vi "Proba.vi"() -> ()   [LabVIEW 2013]
panel:
  out "ora":dbl
  in  "tsim [nap]":i32=7
  in  "h [s]":i32=60
  in  "rhoPCM":dbl=1100.0
  in  "Tbelsolevego_0":dbl=22.0
  in  "c_lev":dbl=1.0
  in  "rholevego":dbl=1.3
  in  "Vlevego":dbl=0.446
  in  "Top_felso":dbl=28.0
  in  "Top_also":dbl=24.0
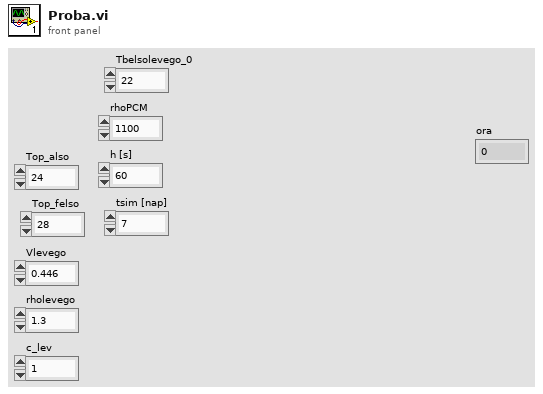
[diagram p1: front panel]
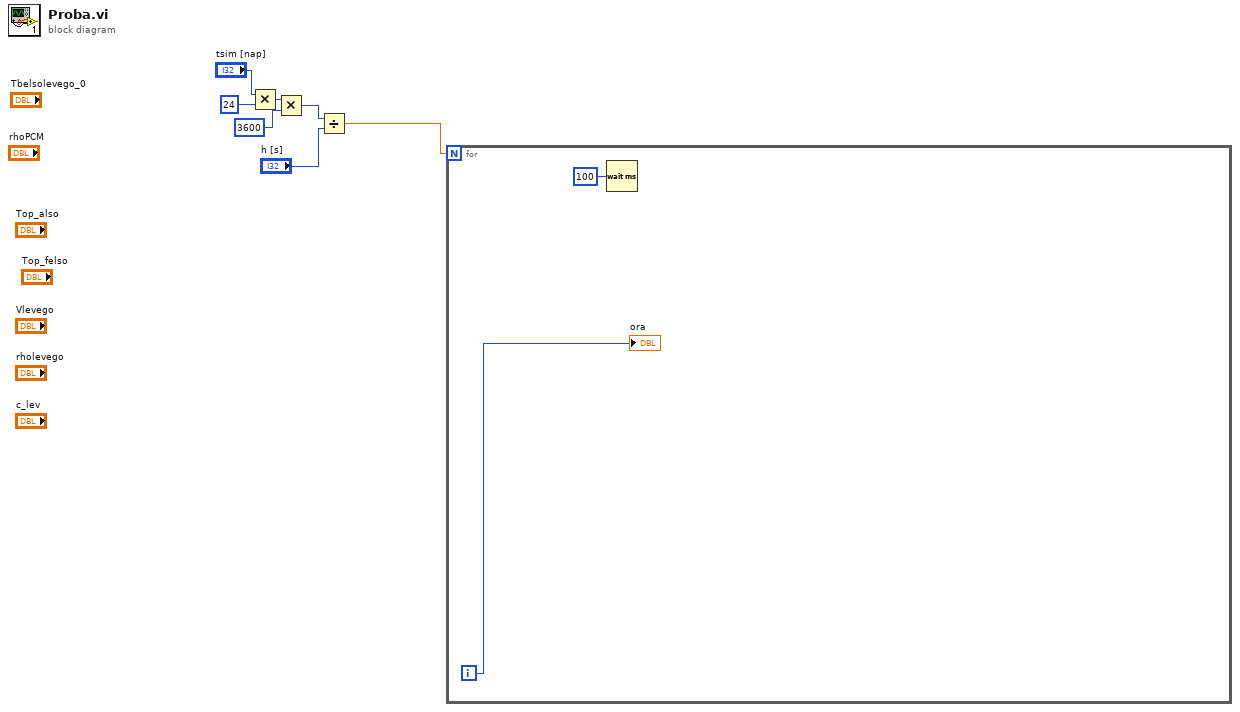
[diagram p0: block diagram]
diagram:
  n1 = Multiply(x="tsim [nap]", y=24) -> (x*y=w5:i32)
  n2 = Multiply(x=w5, y=3600) -> (x*y=w3:i32)
  n3 = Divide(x=w3, y="h [s]") -> (x/y=w1:dbl)
  n4 = for {
    N: w1 -> [_]
    i -> [w8]
    n5 = Wait (ms)(milliseconds to wait=u32 100) -> ()  [unwired: 1 out]
    "ora" <- w8
  }
